vi "Google Earth - Get Co-ords from screen position.vi"(8 "error in":errorcluster, 9 "screen_y":dbl, 10 "screen_x":dbl, 11 "Refnum In":refnum<k7>) -> (0 "error out":errorcluster, 3 "RefnumOut":refnum<k7>)   [LabVIEW 8.6]
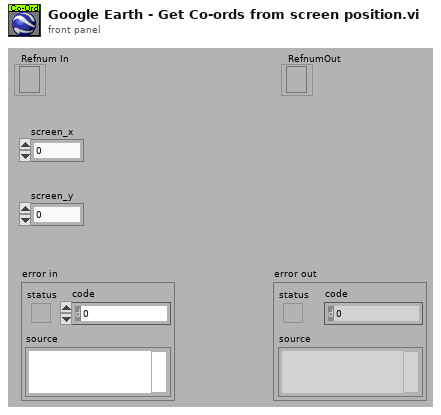
[diagram p1: front panel]
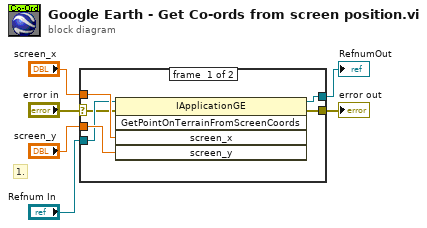
[diagram p0: block diagram]
diagram:
  # "1."
  n1 = case shown="No Error" "error in" {
    selector: "error in" -> [w7 w14]
    tunnel: "screen_y" -> [w12 _]
    tunnel: "screen_x" -> [w11 _]
    tunnel: "Refnum In" -> [w10 w13]
    tunnel: [w9 w13] -> w3
    tunnel: [w8 w14] -> w2
    frame #0 {
      n2 = invoke class="IApplicationGE" method="GetPointOnTerrainFromScreenCoords"(reference=w10, error in=w7, "screen_x"=w11, "screen_y"=w12) -> (reference out=w9:refnum<k7>, error out=w8:errorcluster)  [unwired: 1 in, 3 out]
    }
    frame #1 {
    }
  }
  "error out" <- w2
  "RefnumOut" <- w3
